vi "GetRxPower.vi"(0 "SAVE FILE PATH":path=path "C:/RageATE/Automated Tests/Tetra WAM/DVT/rxdata.csv", 1 "CloseCOM4":bool, 2 "Plot":u16(ring) items=["NoPlot", "PlotAvg", "PlotSamples"], 3 "RunAM_Init":bool=TRUE, 4 "UseFastData(T)":bool=TRUE, 5 "error in (no error)":errorcluster, 6 "dBFS Ofset":dbl, 7 "SAVE TO FILE(T)":bool, 8 "INPUT FILE PATH":path, 9 "INPUT FROM FILE(T)":bool, 11 "CF(MHZ)":dbl=10.0 min=0.0 max=150.0 format="%#_13g", 13 "BW(MHZ)":dbl=10.0 format="%#_13g", 15 "AMInitDyn(t)":bool, 18 "#ofAvg":i32=10) -> (10 "band (dbfs/mhz)":dbl[](array[numeric])=[-40.41732245857817, 9.96580361504641] format="%#_4g", 12 "peak (dbfs/mhz)":dbl[](array[numeric])=[-43.929, 10.039082] format="%#_4g", 14 "Locked?(T)":bool=TRUE, 16 "Am_Init_Flag":bool, 19 "error out":errorcluster={"status"=FALSE, "code"=1073676418, "source"="VISA Close in GetRxPower.vi"})   [LabVIEW 2018]
uses:
  Initialize References/Sequence Globals.vi
  Tetra_Globals.vi
panel:
  out "gui working directory":path=path "C:/TetraLabGUI"
  out "standard error":string
  out "UseAVG(t)":bool
  out "cmd_in":string
  out "standard output":string="2939 49c4\r\n403 6001\r\nFound COM4\r\nseq off\r\nwr reg 0x02 0x0400\r\nwr reg 0x03 0x0000\r\nwr reg 0x04 1032\r\nwr reg 0x05 4\r\nwr reg 0x06 10\r\nwr reg 0x08 256\r\nwr reg 0x09 51\r\nwr reg 0x0A 4\r\nwr reg 0x0E 8000\r\nwr reg 0x0F 0x5555\r\nwr reg 0x10 0x0055\r\nwr reg 0x11 0xAAAA\r\nwr reg 0x12 0x00AA\r\nwr reg 0x1A 0x0000\r\nwr reg 0x1B 0x0000\r\nwr reg 0x17 0x0300\r\nwr reg 0x18 0x0000\r\nsos\r\n"
  out "Time(ms)":u32=1465
  out "start":u32=9009331
  out "console  output":string="b'OK\\n\\r'\r\n[-26 -27 -23 ... -15 -16 -17]\r\nMax Value: -43.929 dBFS at 10.039082 MHz\r\nCF_OUT(MHz) = 9.96580361504641\r\nBP_OUT(dBfs) = -40.41732245857817\r\n"
  # "Input Dialog. Check \"Show Plot\" if desired"
  # "File Path Dialog. Check if file save desired"
  # "Band  & Peak Power Outputs"
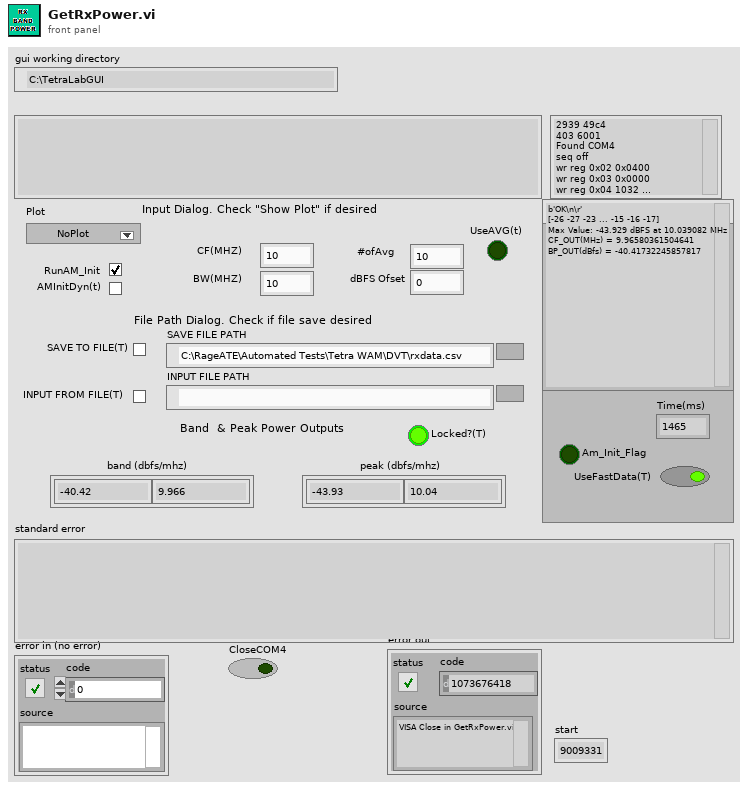
[diagram p1: front panel]
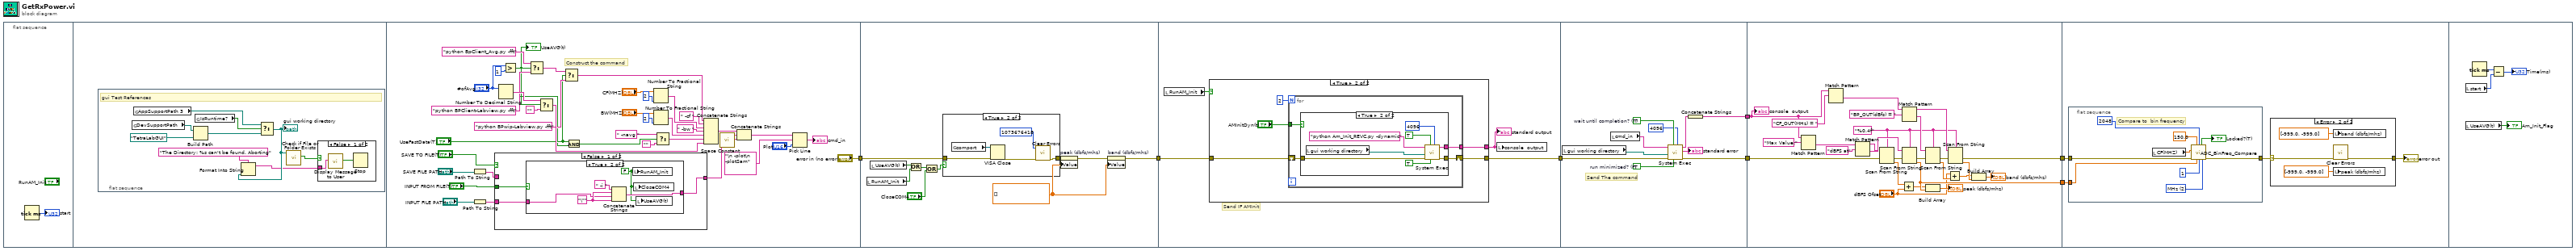
[diagram p0: block diagram]
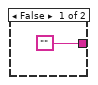
[diagram p3: hidden frame]
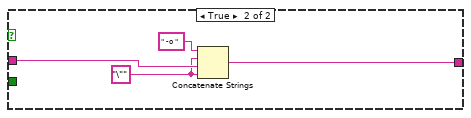
[diagram p4: hidden frame]
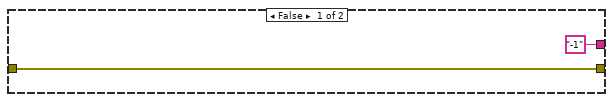
[diagram p6: hidden frame]
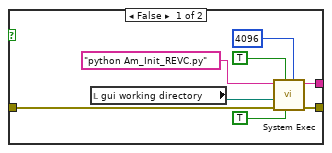
[diagram p7: hidden frame]
diagram:
  n1 = flat-sequence {
    tunnel: ["error in (no error)"] -> w1
    tunnel: [w78] -> w2
    tunnel: w1 -> [w77]
    tunnel: [w90] -> w5
    tunnel: w2 -> [w89]
    tunnel: [w121] -> w7
    tunnel: [w124] -> w6
    tunnel: w5 -> [w123]
    tunnel: w7 -> [w151]
    tunnel: w6 -> [w135]
    tunnel: [w136] -> w4
    tunnel: [w134] -> w3
    tunnel: w4 -> [w157]
    tunnel: w3 -> [w156]
    frame #0 {
      n2 = Tick Count (ms)() -> (millisecond timer value=→"start":u32)
    }
    frame #1 {
      n3 = flat-sequence {
        frame #0 {
          # "gui Test References"
          n4 = global read "Sequence Globals.vi" "DevSupportPath"() -> (w15:path)
          n5 = global read "Sequence Globals.vi" "AppSupportPath 3"() -> (w16:path)
          n6 = Build Path(base path=w15, name or relative path=path "TetraLabGUI" ("gui working directory")) -> (appended path=w13:path)
          n7 = global read "Sequence Globals.vi" "IsRuntime?"() -> (w17:bool)
          n8 = Select(t=w16, s=w17, f=w13) -> (s? t:f=w10:path)
          "gui working directory" <- w10
          n9 = Format Into String(format string="The Directory: %s can't be found. Aborting", w10) -> (resulting string=w9:string)  [unwired: 2 in, 1 out]
          n10 = call <vilib>:"Check if File or Folder Exists.vi"("path"=w10) -> ("file or folder exists?"=w12:bool)  [unwired: 8 in, 2 out]
          n11 = case shown="False" w12 {
            tunnel: w9 -> [w18 _]
            frame False {
              n12 = call "Display Message to User"("Message"=w18) -> ("OK"=w19:bool)  [unwired: 9 in, 1 out]
              n13 = Stop(stop? (T)=w19) -> ()
            }
            frame True {
            }
          }
        }
      }
    }
    frame #2 {
      # "Construct the command"
      n14 = Path To String(path="SAVE FILE PATH") -> (string=w46:string)
      n15 = Path To String(path="INPUT FILE PATH") -> (string=w56:string)
      n16 = case shown="False" "SAVE TO FILE(T)" {
        tunnel: w46 -> [_ w70]
        tunnel: [w60 w69] -> w54
        tunnel: w56 -> [w59 _]
        tunnel: "INPUT FROM FILE(T)" -> [w58 _]
        frame False {
          n17 = case shown="True" w58 {
            tunnel: ["" w64] -> w60
            tunnel: w59 -> [_ w63]
            frame False {
            }
            frame True {
              w62 = FALSE ("RunAM_Init")
              w65 = "\"" ("string")
              n18 = Concatenate Strings(" -i " ("string"), w65, w63, w65) -> (w64:string)
              n19 = local write "RunAM_Init"(w62) -> ()
              n20 = local write "CloseCOM4"(w62) -> ()
              n21 = local write "UseAVG(t)"(w62) -> ()
            }
          }
        }
        frame True {
          w67 = "\"" ("string")
          n22 = Concatenate Strings(" -o " ("string"), w67, w70, w67) -> (w69:string)
        }
      }
      n23 = Number To Decimal String(number="#ofAvg") -> (decimal integer string=w42:string)  [unwired: 1 in]
      n24 = Greater?(x="#ofAvg", y=1 ("x")) -> (0:w27:bool)
      "UseAVG(t)" <- w27
      n25 = Select(t="python BpClient_Avg.py -fft" ("command line"), s=w27, f="python BPClient-Labview.py -fft" ("command line")) -> (s? t:f=w34:string)
      n26 = Select(t=w42, s=w27, f="") -> (s? t:f=w43:string)
      n27 = Select(t=w34, s="UseFastData(T)", f="python BPwip-Labview.py -fft" ("command line")) -> (s? t:f=w32:string)
      n28 = And(x="UseFastData(T)", y=w27) -> (x .and. y?=w26:bool)
      n29 = Number To Fractional String(number="CF(MHZ)", precision (6)=i16 2) -> (F-format string=w50:string)  [unwired: 2 in]
      n30 = Number To Fractional String(number="BW(MHZ)", precision (6)=i16 2) -> (F-format string=w51:string)  [unwired: 2 in]
      n31 = Select(t=" -navg " ("string"), s=w26, f="") -> (s? t:f=w39:string)
      n32 = Concatenate Strings(w32, " -cf " ("string"), w50, " -bw " ("string"), w51, w39, w43) -> (w52:string)
      n33 = call <vilib>:"Space Constant.vi"() -> ("String"=w21:string)
      n34 = Concatenate Strings(w52, w54, w21) -> (w23:string)
      n35 = Pick Line(string ("")=w23, multi-line string="\n -plot\n -plotSam", line index="Plot") -> (output string=→"cmd_in":string)
    }
    frame #3 {
      w79 = dbl[] [] ("peak (dbfs/mhz)")
      n36 = local read "RunAM_Init"() -> (w74:bool)
      n37 = local read "UseAVG(t)"() -> (w71:bool)
      n38 = Or(x=w71, y=w74) -> (x .or. y?=w75:bool)
      n39 = Or(x=w75, y="CloseCOM4") -> (x .or. y?=w72:bool)
      n40 = case shown="True" w72 {
        tunnel: w77 -> [w81 w85]
        tunnel: [w81 w82] -> w76
        frame False {
        }
        frame True {
          n41 = global read "Tetra_Globals.vi" "comport"() -> (w86:refnum<visa-resource-name>)
          n42 = VISA Close(VISA resource name=w86, error in (no error)=w85) -> (error out=w83:errorcluster)
          n43 = call <vilib>:"Clear Errors.vi"("error in (no error)"=w83, "specific error code to clear (0: all)"=1073676418) -> ("error out"=w82:errorcluster)  [unwired: 4 in, 1 out]
        }
      }
      n44 = property on="peak (dbfs/mhz)" class="Arr (strict)"(error in=w76, "Value"=w79) -> (error out=w80:errorcluster)  [unwired: 1 in, 1 out]
      n45 = property on="band (dbfs/mhz)" class="Arr (strict)"(error in=w80, "Value"=w79) -> (error out=w78:errorcluster)  [unwired: 1 in, 1 out]
    }
    frame #4 {
      # "Send IF AMInit"
      n46 = local read "RunAM_Init"() -> (w88:bool)
      n47 = case shown="True" w88 {
        tunnel: [w92 w97] -> w90
        tunnel: w89 -> [w92 w96]
        tunnel: ["-1" ("standard output") w95] -> w87
        frame False {
        }
        frame True {
          n48 = for {
            N: 2 -> [_]
            tunnel: [w99] -> w95
            tunnel: "AMInitDyn(t)" -> [w98]
            shift-right: [w101] -> w97
            shift-left: w96 -> [w100]
            n49 = case shown="True" w98 {
              tunnel: [w108 w116] -> w101
              tunnel: w100 -> [w105 w113]
              tunnel: [w104 w112] -> w99
              frame False {
                n50 = local read "gui working directory"() -> (w102:path)
                n51 = call <vilib>:"System Exec.vi"("expected output size  (4096)"=u32 4096, "run minimized? (F)"=TRUE, "wait until completion? (T)"=TRUE, "error in (no error)"=w105, "working directory"=w102, "command line"="python Am_Init_REVC.py") -> ("error out"=w108:errorcluster, "standard output"=w104:string)  [unwired: 2 in, 2 out]
              }
              frame True {
                n52 = local read "gui working directory"() -> (w110:path)
                n53 = call <vilib>:"System Exec.vi"("expected output size  (4096)"=u32 4096, "run minimized? (F)"=TRUE, "wait until completion? (T)"=TRUE, "error in (no error)"=w113, "working directory"=w110, "command line"="python Am_Init_REVC.py -dynamic") -> ("error out"=w116:errorcluster, "standard output"=w112:string)  [unwired: 2 in, 2 out]
              }
            }
          }
        }
      }
      "standard output" <- w87
      n54 = local write "console  output"(w87) -> ()
    }
    frame #5 {
      w126 = TRUE  # wait until completion? (T)
      w127 = TRUE  # run minimized? (F)
      # "Send The command"
      n55 = local read "gui working directory"() -> (w118:path)
      n56 = local read "cmd_in"() -> (w119:string)
      n57 = call <vilib>:"System Exec.vi"("expected output size  (4096)"=u32 4096, "run minimized? (F)"=w127, "wait until completion? (T)"=w126, "error in (no error)"=w123, "working directory"=w118, "command line"=w119) -> ("error out"=w124:errorcluster, "standard error"=→"standard error":string, "standard output"=w125:string)  [unwired: 2 in, 1 out]
      n58 = Concatenate Strings(w125) -> (w121:string)
    }
    frame #6 {
      w140 = "%0.4f" ("format string")
      n59 = Match Pattern(string=w151, regular expression="Max Value:") -> (after substring=w147:string)  [unwired: 1 in, 3 out]
      n60 = Match Pattern(string=w151, regular expression="CF_OUT(MHz) = ") -> (after substring=w143:string)  [unwired: 1 in, 3 out]
      n61 = Match Pattern(string=w147, regular expression="dBFS at") -> (before substring=w148:string, after substring=w149:string)  [unwired: 1 in, 2 out]
      n62 = Scan From String(format string=w140, input string=w148, error in=w135) -> (error out=w133:errorcluster, output 1=w152:dbl)  [unwired: 2 in, 2 out]
      n63 = Add(x=w152, y="dBFS Ofset") -> (x+y=w130:dbl)
      n64 = Match Pattern(string=w143, regular expression="BP_OUT(dBfs) = ") -> (before substring=w142:string, after substring=w141:string)  [unwired: 1 in, 2 out]
      n65 = Scan From String(format string=w140, input string=w149, error in=w133) -> (error out=w132:errorcluster, output 1=w136:dbl)  [unwired: 2 in, 2 out]
      n66 = Scan From String(format string=w140, input string=w141, error in=w132) -> (error out=w131:errorcluster, output 1=w138:dbl)  [unwired: 2 in, 2 out]
      n67 = Build Array(w130, w136) -> (→"peak (dbfs/mhz)":dbl[])
      n68 = Add(x="dBFS Ofset", y=w138) -> (x+y=w129:dbl)
      n69 = Scan From String(format string=w140, input string=w142, error in=w131) -> (error out=w134:errorcluster, output 1=w137:dbl)  [unwired: 2 in, 2 out]
      n70 = Build Array(w129, w137) -> (→"band (dbfs/mhz)":dbl[])
      "console  output" <- w151
    }
    frame #7 {
      n71 = flat-sequence {
        tunnel: [w170] -> w155
        tunnel: w156 -> [w166]
        tunnel: w157 -> [w165]
        frame #0 {
          w167 = u16 2 items=["Hz", "KHz", "MHz"] ("F units")
          # "Compare to  bin frequency"
          n72 = local read "CF(MHZ)"() -> (w163:dbl)
          n73 = call "ADC_BinFreq_Compare.vi"("Fsample"=150.0, "# of Samples"=2048, "Expected Frequency"=w163, "error in"=w166, "Input Freq"=w165, "+/- error(bins)"=1, "F units"=w167) -> ("In Range?(T)"=→"Locked?(T)":bool, "error out"=w170:errorcluster)  [unwired: 6 in, 1 out]
        }
      }
      n74 = case shown="Error" w155 {
        selector: w155 -> [w158 w160]
        tunnel: [w158 w159] -> w154
        frame No Error {
        }
        frame Error {
          n75 = local write "band (dbfs/mhz)"(dbl[] [-999.0, -999.0] ("band (dbfs/mhz)")) -> ()
          n76 = call <vilib>:"Clear Errors.vi"("error in (no error)"=w160) -> ("error out"=w159:errorcluster)  [unwired: 5 in, 1 out]
          n77 = local write "peak (dbfs/mhz)"(dbl[] [-999.0, -999.0] ("peak (dbfs/mhz)")) -> ()
        }
      }
      "error out" <- w154
    }
    frame #8 {
      n78 = local read "start"() -> (w174:u32)
      n79 = local read "UseAVG(t)"() -> (→"Am_Init_Flag":bool)
      n80 = Tick Count (ms)() -> (millisecond timer value=w175:u32)
      n81 = Subtract(x=w175, y=w174) -> (x-y=→"Time(ms)":u32)
    }
  }
